vi "sub_joystick-data-conv_remote.vi"(11 "joystick info-in":T1) -> (2 "cmd":u32, 3 "opval":cluster{dbl, dbl} {"?" format="%-1.1f"; "?" format="%-1.1f"})   [LabVIEW 2019]
uses:
  Ctrl/cmd_common.ctl
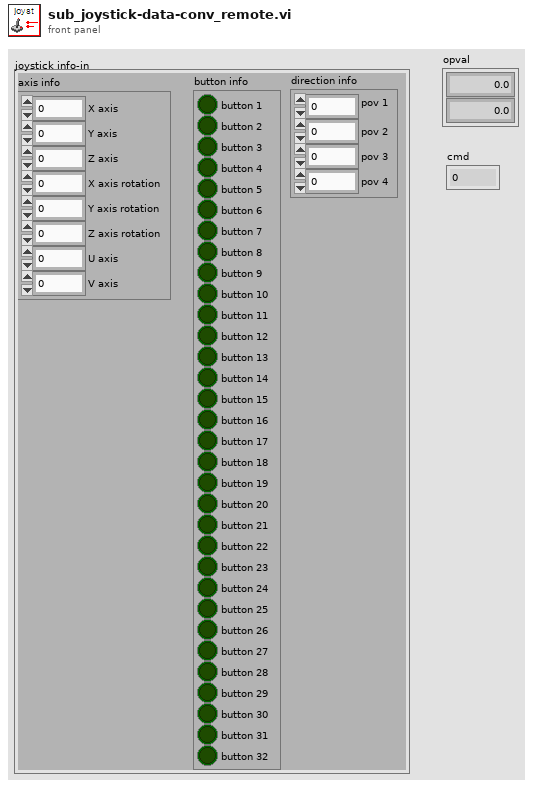
[diagram p1: front panel]
types:
  T1 = cluster{"axis info":cluster{"X axis":i32, "Y axis":i32, "Z axis":i32, "X axis rotation":i32, "Y axis rotation":i32, "Z axis rotation":i32, "U axis":i32, "V axis":i32}, "button info":cluster{"button 1":bool, "button 2":bool, "button 3":bool, "button 4":bool, "button 5":bool, "button 6":bool, "button 7":bool, "button 8":bool, "button 9":bool, "button 10":bool, "button 11":bool, "button 12":bool, "button 13":bool, "button 14":bool, "button 15":bool, "button 16":bool, "button 17":bool, "button 18":bool, "button 19":bool, "button 20":bool, "button 21":bool, "button 22":bool, "button 23":bool, "button 24":bool, "button 25":bool, "button 26":bool, "button 27":bool, "button 28":bool, "button 29":bool, "button 30":bool, "button 31":bool, "button 32":bool}, "direction info":cluster{"pov 1":i32, "pov 2":i32, "pov 3":i32, "pov 4":i32}}
  T2 = enum16{"none", "ERP42", "ERP42mini", "Scout", "Ycar"}
  T3 = typedef "cmd_common.ctl" = enum16{"read", "write"}
  T4 = typedef "joystick cfg.ctl" = cluster{"Type":enum16{"Logitech F710", "Xbox"}, "steer limit":cluster{"min":dbl, "max":dbl, "scale":dbl, "offset":dbl}, "speed limit":cluster{"min":dbl, "max":dbl, "pwm max":dbl}, "ID":i32, "joystick max":dbl}
  T5 = cluster{"button 1":bool, "button 2":bool, "button 3":bool, "button 4":bool, "button 5":bool, "button 6":bool, "button 7":bool, "button 8":bool, "button 9":bool, "button 10":bool, "button 11":bool, "button 12":bool, "button 13":bool, "button 14":bool, "button 15":bool, "button 16":bool, "button 17":bool, "button 18":bool, "button 19":bool, "button 20":bool, "button 21":bool, "button 22":bool, "button 23":bool, "button 24":bool, "button 25":bool, "button 26":bool, "button 27":bool, "button 28":bool, "button 29":bool, "button 30":bool, "button 31":bool, "button 32":bool}
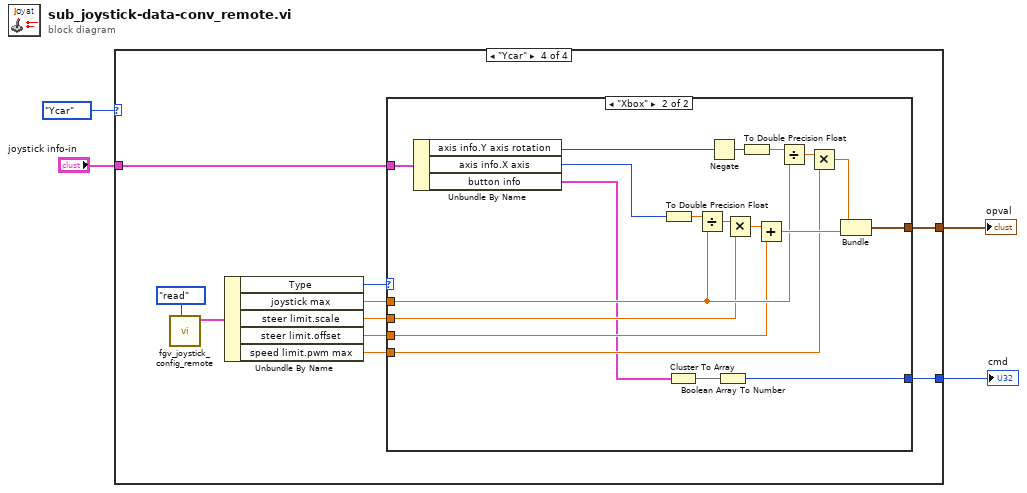
[diagram p0: block diagram]
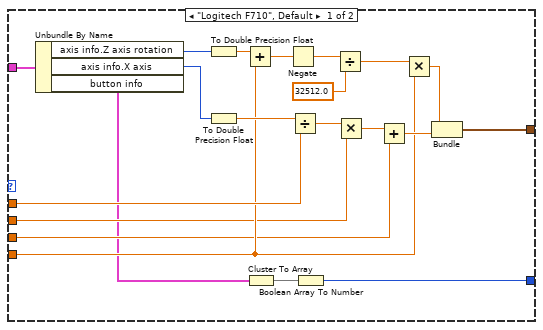
[diagram p5: hidden frame]
diagram:
  n1 = case shown="\"Ycar\"" T2."Ycar" ("AGV") {
    tunnel: [_ _ _ w14] -> w4
    tunnel: "joystick info-in" -> [_ _ _ w13]
    tunnel: [_ _ _ w8] -> w1
    frame "ERP42", Default {
    }
    frame "ERP42mini" {
    }
    frame "Scout" {
    }
    frame "Ycar" {
      n2 = call "fgv_joystick_config_remote.vi"("cmd"=cmd_common."read") -> ("Joystick cfg out"=w6:T4)  [unwired: 9 in, 1 out]
      n3 = Unbundle By Name(w6) -> ("Type"=w7:enum16{"Logitech F710", "Xbox"}, "joystick max"=w12:dbl, "steer limit.scale"=w11:dbl, "steer limit.offset"=w10:dbl, "speed limit.pwm max"=w9:dbl)
      n4 = case shown="\"Xbox\"" w7 {
        tunnel: [w35 w45] -> w14
        tunnel: w13 -> [w25 w47]
        tunnel: w12 -> [w21 w42]
        tunnel: w11 -> [w19 w41]
        tunnel: w10 -> [w18 w40]
        tunnel: w9 -> [w20 w39]
        tunnel: [w15 w36] -> w8
        frame "Logitech F710", Default {
          n5 = Unbundle By Name(w25) -> ("axis info.Z axis rotation"=w24:i32, "axis info.X axis"=w30:i32, "button info"=w16:T5)
          n6 = To Double Precision Float(number=w24) -> (double precision float=w27:dbl)
          n7 = To Double Precision Float(number=w30) -> (double precision float=w26:dbl)
          n8 = Add(x=w27, y=w20) -> (x+y=w34:dbl)
          n9 = Cluster To Array(cluster=w16) -> (array=w17:bool[])
          n10 = Negate(x=w34) -> (-x=w32:dbl)
          n11 = Divide(x=w26, y=w21) -> (x/y=w29:dbl)
          n12 = Boolean Array To Number(Boolean array=w17) -> (number=w15:u32)
          n13 = Divide(x=w32, y=32512.0) -> (x/y=w31:dbl)
          n14 = Multiply(x=w29, y=w19) -> (x*y=w28:dbl)
          n15 = Add(x=w28, y=w18) -> (x+y=w22:dbl)
          n16 = Multiply(x=w31, y=w20) -> (x*y=w23:dbl)
          n17 = Bundle(w23, w22) -> (w35:cluster{dbl, dbl})  [unwired: 1 in]
        }
        frame "Xbox" {
          n18 = Unbundle By Name(w47) -> ("axis info.Y axis rotation"=w48:i32, "axis info.X axis"=w54:i32, "button info"=w38:T5)
          n19 = To Double Precision Float(number=w54) -> (double precision float=w51:dbl)
          n20 = Cluster To Array(cluster=w38) -> (array=w37:bool[])
          n21 = Divide(x=w51, y=w42) -> (x/y=w53:dbl)
          n22 = Negate(x=w48) -> (-x=w46:i32)
          n23 = Boolean Array To Number(Boolean array=w37) -> (number=w36:u32)
          n24 = Multiply(x=w53, y=w41) -> (x*y=w52:dbl)
          n25 = To Double Precision Float(number=w46) -> (double precision float=w50:dbl)
          n26 = Add(x=w52, y=w40) -> (x+y=w43:dbl)
          n27 = Divide(x=w50, y=w42) -> (x/y=w49:dbl)
          n28 = Multiply(x=w49, y=w39) -> (x*y=w44:dbl)
          n29 = Bundle(w44, w43) -> (w45:cluster{dbl, dbl})  [unwired: 1 in]
        }
      }
    }
  }
  "opval" <- w4
  "cmd" <- w1
